vi "SrvUnregisterArea.vi"(0 "ref in":u64, 5 "AreaCode":i32(ring)=5 items=["Inputs (EB)", "Output (AB)", "Bit Memory (M)", "Counters (Z)", "Timers (T)", "Data (DB)"], 7 "Index":u16=1, 11 "error in (no error)":errorcluster) -> (4 "ref out":u64, 6 "Result":i32, 15 "error out":errorcluster)   [LabVIEW 2020, in "Snap7.lvlib"]
uses:
  Snap7.lvlib
  windows/lv_snap7.dll
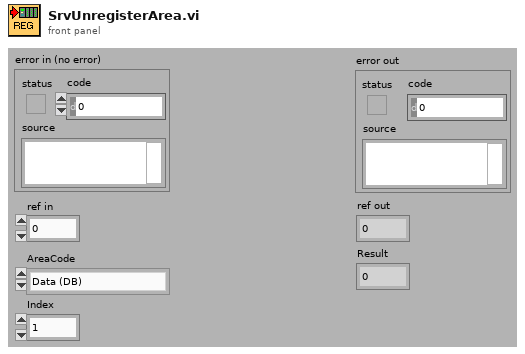
[diagram p1: front panel]
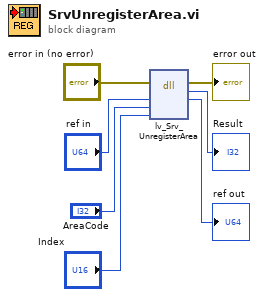
[diagram p0: block diagram]
diagram:
  n1 = dll-call lib="PTH2fabs CUsersFeng项目HLCEPS300-2性能试验台SourcesSnap7libwindowslv_snap7.dll" fn="lv_Srv_UnregisterArea"(error in="error in (no error)", "Server"="ref in", "Area"="AreaCode", "Index"="Index") -> (error out=→"error out":errorcluster, "return type"=→"Result":i32, "Server"=→"ref out":u64)  [unwired: 4 in, 1 out]
